vi "Read Test Group Manager.vi"(8 "error in (no error)":errorcluster, 11 "Measurement Interface in":refnum<class "Measurement Interface.lvclass">) -> (0 "error out":errorcluster, 2 "Test Group Manager":refnum<data-value>, 3 "Measurement Interface out":refnum<class "Measurement Interface.lvclass">)   [LabVIEW 2016, in "Measurement Interface.lvlib" / "Measurement Interface.lvclass"]
uses:
  Measurement Interface.lvclass
  Plugins/Test Group Manager.lvlibp/Test Group Manager.lvclass
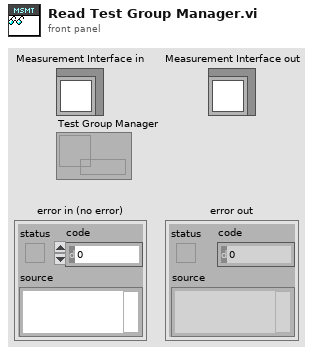
[diagram p1: front panel]
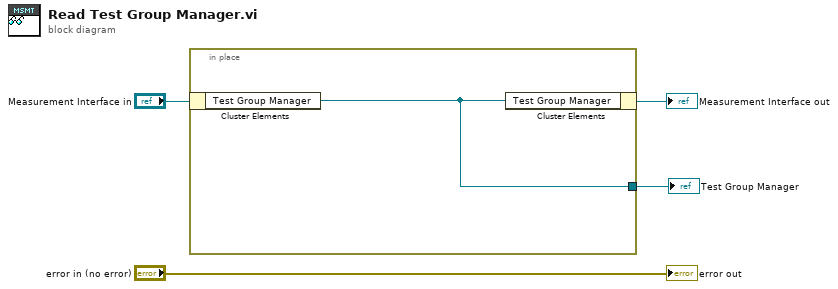
[diagram p0: block diagram]
diagram:
  n1 = in-place {
    in-place-border: [w5] -> w2
    n2 = in-place-cluster #1("Measurement Interface in") -> ("Test Group Manager"=w5:refnum<data-value>)
    n3 = in-place-cluster #1("Test Group Manager"=w5) -> (→"Measurement Interface out":refnum<class "Measurement Interface.lvclass">)
  }
  "Test Group Manager" <- w2
  "error out" <- "error in (no error)"
